vi "Draw Gradient Circle.vi"(5 "arc size(360)":i16=360 caption="圆弧大小(360)", 7 "start angle(0)":i16 caption="起始角(0)", 8 "Color Segement":u32[](array[colorbox])=[16448250, 0], 9 "pixel center":cluster{"horizontal":i16, "vertical":i16}={"horizontal"=100, "vertical"=100} caption="Circle Center", 10 "radius":i16=100, 11 "picture in":picture) -> (3 "picture out":picture)   [LabVIEW 2012, in "Gradient PieChart.lvclass"]
uses:
  Gradient PieChart.lvclass
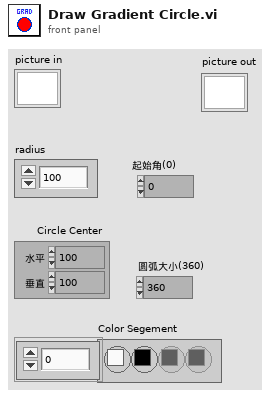
[diagram p1: front panel]
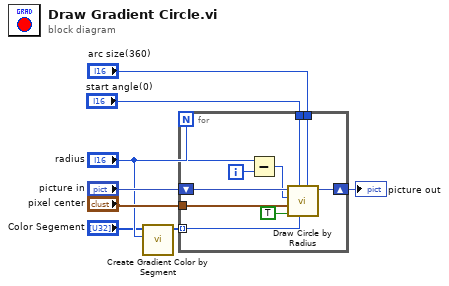
[diagram p0: block diagram]
diagram:
  n1 = call "Create Gradient Color by Segment.vi"("Length"="radius", "Color Segement"="Color Segement") -> ("1 Pix H - Color Box Array"=w7:u32[])  [unwired: 7 in, 2 out]
  n2 = for {
    N: "radius" -> [w14]
    tunnel: "pixel center" -> [w18]
    tunnel: w7 -> [w17] mode=indexing
    shift-right: [w16] -> w6
    shift-left: "picture in" -> [w15]
    tunnel: "start angle(0)" -> [w10]
    tunnel: "arc size(360)" -> [w9]
    i -> [w13]
    n3 = Subtract(x=w14, y=w13) -> (x-y=w12:i32)
    n4 = call <vilib>:"Draw Circle by Radius.vi"("arc size(360)"=w9, "color(black)"=w17, "start angle(0)"=w10, "fill?(F)"=TRUE, "pixel center"=w18, "radius"=w12, "picture"=w15) -> ("new picture"=w16:picture)  [unwired: 4 in]
  }
  "picture out" <- w6
